vi "RunMe.vi"   [LabVIEW 2019]
uses:
  <userlib>/LevyLab/Build Support/ProjectItem/API/Instrument Name and Icon UI.vi
  <userlib>/LevyLab/Build Support/ProjectItem/ProjectItem.lvclass
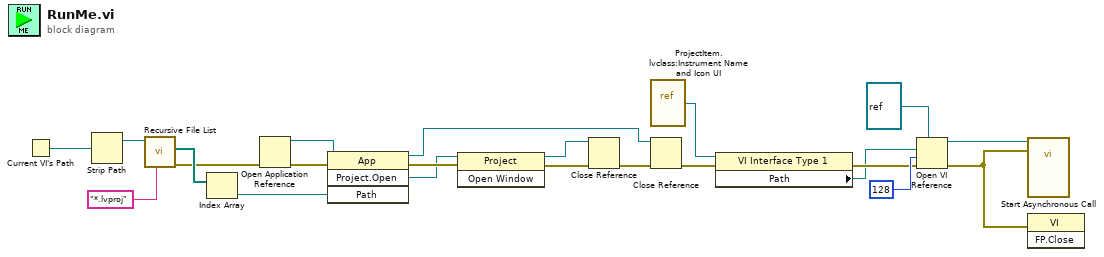
[diagram p0: block diagram]
diagram:
  n1 = Current VI's Path() -> (path=w22:path)
  n2 = Strip Path(path=w22) -> (stripped path=w21:path)  [unwired: 1 out]
  n3 = call <vilib>:"Recursive File List.vi"("pattern"="*.lvproj", "Folder Path"=w21) -> ("error out"=w7:errorcluster, "All Files in Dir"=w19:path[])  [unwired: 5 in, 3 out]
  n4 = Index Array(array=w19) -> (element=w15:path)  [unwired: 1 in]
  n5 = Open Application Reference(8:w7) -> (0:w13:errorcluster, 3:w16:refnum<vi>)  [unwired: 3 in]
  n6 = invoke class="App" method="Project.Open"(reference=w16, error in=w13, "Path"=w15) -> (reference out=w11:refnum<vi>, error out=w14:errorcluster, "Project:Open"=w12:refnum<vi>)  [unwired: 1 in, 1 out]
  n7 = invoke class="Project" method="Open Window"(reference=w12, error in=w14) -> (reference out=w18:refnum<vi>, error out=w17:errorcluster)  [unwired: 1 in, 1 out]
  n8 = Close Reference(reference=w18, error in (no error)=w17) -> (error out=w10:errorcluster)
  n9 = vi-ref "ProjectItem.lvclass:Instrument Name and Icon UI.vi"() -> (w4:refnum<vi>)
  n10 = Close Reference(reference=w11, error in (no error)=w10) -> (error out=w3:errorcluster)
  n11 = property class="VI Interface Type 1"(reference=w4, error in=w3) -> (error out=w2:errorcluster, "Path"=w1:path)  [unwired: 1 out]
  n12 = Open VI Reference(type specifier VI Refnum (for type only)=refnum<vi> refnum, vi path=w1, options=128, error in (no error)=w2) -> (vi reference=w6:refnum<vi>, error out=w8:errorcluster)  [unwired: 2 in]
  n13 = call-by-ref "Start Asynchronous Call"(reference=w6, error in=w8) -> ()  [unwired: 12 in, 2 out]
  n14 = invoke class="VI" method="FP.Close"(error in=w8) -> ()  [unwired: 2 in, 3 out]
